vi "Read Event Registration.vi"(7 "subchannel":i32, 10 "channel":T1) -> (2 "event registration refnum":refnum<event-registration>)   [LabVIEW 2019, in "Event MessengerM.lvlib"]
doc: "<p>Reads an <a href=\"nihelplauncher://docs/csh?context=lvcore_lvconcepts_using_events_in_labview\">event registration</a> refnum for an Event Messenger <a href=\"nihelplauncher://docs/csh?context=lvcore_lvconcepts_channel_wires_intro\">channel</a>.</p>"
uses:
  Event MessengerM.lvlib
  <resource>/ChannelSupport/_ChannelSupport/GetErrors/FpgaChannelWireNotSupported.xnode
  ChannelOp.ctl
  ))Channel.ctl
  Event Data.ctl
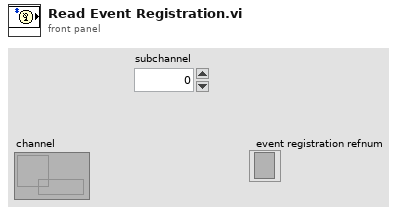
[diagram p1: front panel]
types:
  T1 = typedef "Event MessengerM.lvlib/))Channel.ctl" = refnum<queue>
  T2 = typedef "Event MessengerM.lvlib/ChannelOp.ctl" = enum16{"init", "write", "register", "replicate", "probe"}
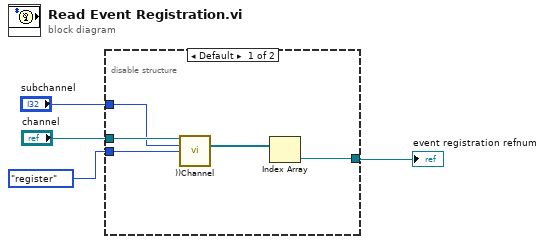
[diagram p0: block diagram]
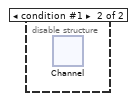
[diagram p2: hidden frame]
diagram:
  n1 = disable-structure shown="Default" {
    disable-tunnel: ChannelOp."register" ("channelOp") -> [w5 _]
    disable-tunnel: "channel" -> [w8 _]
    disable-tunnel: [w9 _] -> w1
    disable-tunnel: "subchannel" -> [w6 _]
    frame condition #0 (active) {
      n2 = call "))Channel.vi"("channel in"=w8, "subchannel"=w6, "channelOp"=w5) -> ("event registration refnums"=w7:refnum<event-registration>[])  [unwired: 8 in, 4 out]
      n3 = Index Array(array=w7) -> (element=w9:refnum<event-registration>)  [unwired: 1 in]
    }
    frame condition #1 {
      n4 = xnode "Channel"() -> ()
    }
  }
  "event registration refnum" <- w1
